vi "Server.vi"(8 "error in":errorcluster) -> (0 "error out":errorcluster, 3 "Received Data":dbl[](array[numeric]))   [LabVIEW 2019]
uses:
  <vilib>/regexp/Match Regular Expression.xnode
panel:
  out "Received Data":cluster{dbl, dbl}(graph)
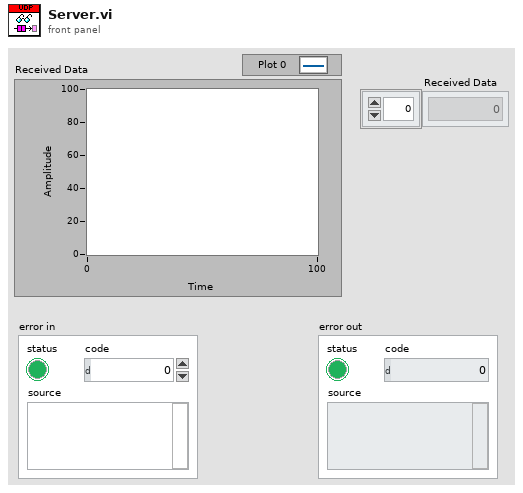
[diagram p1: front panel]
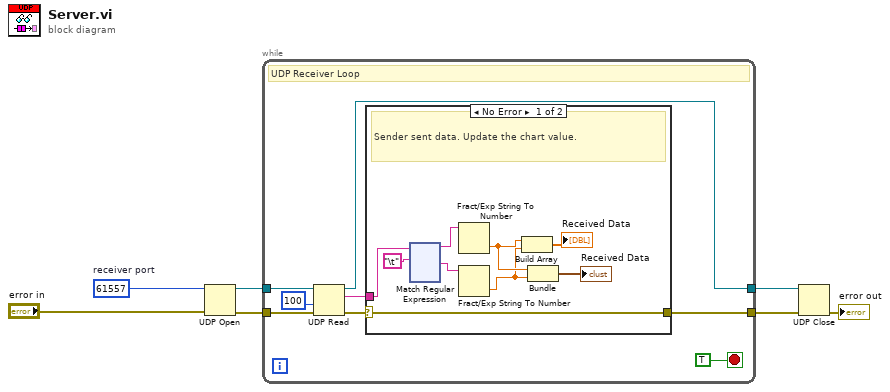
[diagram p0: block diagram]
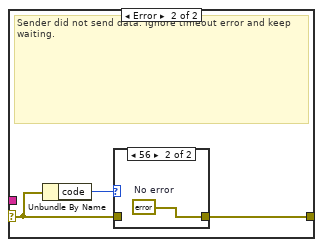
[diagram p2: hidden frame]
diagram:
  w3 = u16 61557  # receiver port
  n1 = UDP Open(8:"error in", 11:w3) -> (port=w4:refnum<k16>, 0:w5:errorcluster)  [unwired: 3 in, 1 out]
  n2 = while {
    tunnel: w4 -> [w15]
    tunnel: [w9] -> w7
    tunnel: w5 -> [w14]
    tunnel: [w10] -> w6
    stop <- TRUE stop-if-true
    # "UDP Receiver Loop"
    n3 = UDP Read(connection ID=w15, timeout ms (25000)=100, 8:w14) -> (data out=w12:string, error out=w11:errorcluster, 3:w9:refnum<k16>)  [unwired: 3 out]
    n4 = case shown="No Error" w11 {
      selector: w11 -> [w24 w140]
      tunnel: w12 -> [w22 _]
      tunnel: [w24 w139] -> w10
      frame No Error {
        # "Sender sent data. Update the chart value."
        n5 = xnode "Match Regular Expression"("input string"=w22, "regular expression"="\t") -> ("before match"=w21:string, "after match"=w20:string)  [unwired: 4 in, 3 out]
        n6 = Fract/Exp String To Number(string=w21) -> (number=w18:dbl)  [unwired: 3 in, 1 out]
        n7 = Fract/Exp String To Number(string=w20) -> (number=w17:dbl)  [unwired: 3 in, 1 out]
        n8 = Build Array(w18, w17) -> (→"Received Data":dbl[])
        n9 = Bundle(w18, w17) -> (→"Received Data":cluster{dbl, dbl})  [unwired: 1 in]
      }
      frame Error {
        # "Sender did not send data. Ignore timeout error and keep waiting."
        n10 = Unbundle By Name(w140) -> ("code"=w141:i32)
        n11 = case shown="56" w141 {
          tunnel: w140 -> [w142 _]
          tunnel: [w142 w143] -> w139
          frame Default {
          }
          frame 56 {
            w143 = errorcluster {"status"=FALSE, "code"=0, "source"=""}  # No error
          }
        }
      }
    }
  }
  n12 = UDP Close(connection ID=w7, 8:w6) -> (error out=→"error out":errorcluster)  [unwired: 1 out]
